vi "LVClass_HasoData Write HasoData ptr create.vi"(8 "error in (no error)":errorcluster, 10 "Enum":T1, 11 "HasoData in":refnum<class "HasoData.lvclass">) -> (0 "error out":errorcluster, 3 "HasoData out":refnum<class "HasoData.lvclass">)   [LabVIEW 2020, in "HasoData.lvclass"]
uses:
  HasoData.lvclass
  Handle creation.ctl
  HasoData.lvclass/HasoData.ctl
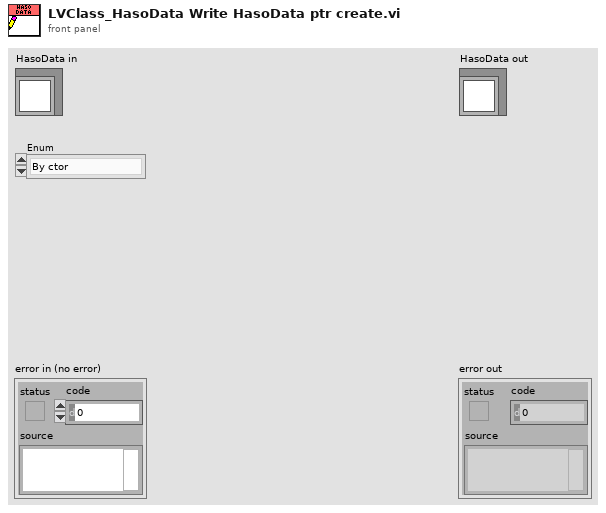
[diagram p1: front panel]
types:
  T1 = typedef "Handle creation.ctl" = enum16{"By ctor", "By write function"}
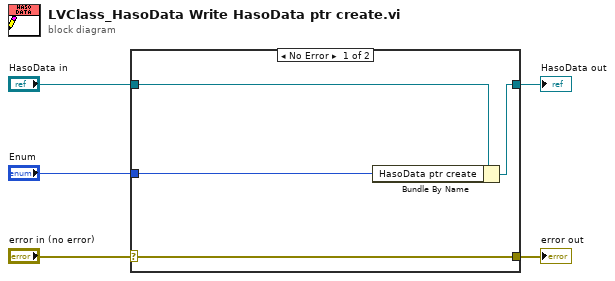
[diagram p0: block diagram]
diagram:
  n1 = case shown="No Error" "error in (no error)" {
    selector: "error in (no error)" -> [w9 w10]
    tunnel: [w9 w10] -> w4
    tunnel: [w7 w11] -> w2
    tunnel: "HasoData in" -> [w8 w11]
    tunnel: "Enum" -> [w6 _]
    frame No Error {
      n2 = Bundle By Name(cluster=w8, "HasoData ptr create"=w6) -> (w7:refnum<class "HasoData.lvclass">)
    }
    frame Error {
    }
  }
  "error out" <- w4
  "HasoData out" <- w2
